vi "FTW-Endpoint-BindToListener.vi"(0 "FTW-Endpoint In":refnum<class "FTW-Endpoint.lvclass">, 5 "Address":string, 9 "Timeout":i32=1000 format="%dmsec", 11 "error in":errorcluster) -> (4 "FTW-Endpoint Out":refnum<class "FTW-Endpoint.lvclass">, 6 "Actual Address":string, 15 "error out":errorcluster)   [LabVIEW 2013, in "FTW-Endpoint.lvclass"]
uses:
  FTW-Endpoint.lvclass
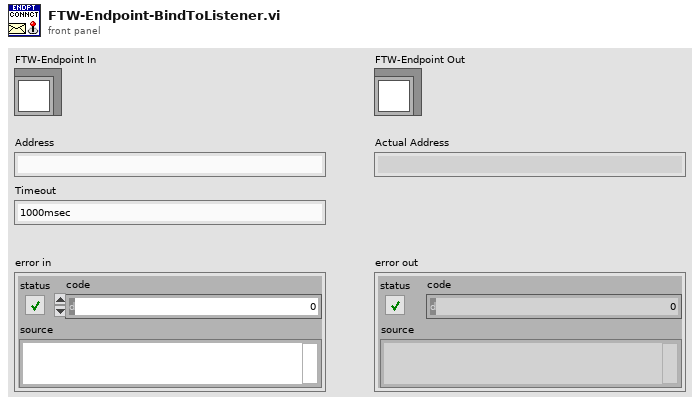
[diagram p1: front panel]
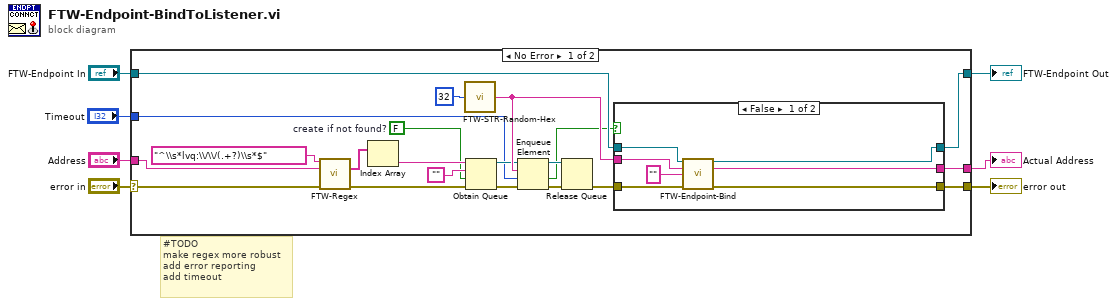
[diagram p0: block diagram]
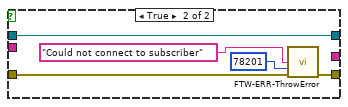
[diagram p2: hidden frame]
diagram:
  # "#TODO\nmake regex more robust\nadd error reporting\nadd timeout"
  n1 = case shown="No Error" "error in" {
    selector: "error in" -> [w26 w42]
    tunnel: [w22 w42] -> w7
    tunnel: [w21 w41] -> w6
    tunnel: "FTW-Endpoint In" -> [w27 w41]
    tunnel: "Address" -> [w18 _]
    tunnel: [w19 _] -> w2
    tunnel: "Timeout" -> [w9 _]
    frame No Error {
      w11 = FALSE  # create if not found?
      n2 = call "FTW-Regex.vi"("Regular Expression"="^\\s*lvq:\\/\\/(.+?)\\s*$" ("input string"), "Input String"=w18, "error in"=w26) -> ("Submatches"=w24:string[], "error out"=w25:errorcluster)  [unwired: 8 in, 3 out]
      n3 = Index Array(array=w24) -> (element=w23:string)  [unwired: 1 in]
      n4 = call "FTW-STR-Random-Hex.vi"("String Length"=32) -> ("Random Hex String"=w20:string)  [unwired: 3 in]
      n5 = Obtain Queue(name (unnamed)=w23, element data type="", create if not found? (T)=w11, error in (no error)=w25) -> (queue out=w14:refnum<queue>, error out=w16:errorcluster)  [unwired: 1 in, 1 out]
      n6 = Enqueue Element(queue=w14, element=w20, timeout in ms (-1)=w9, error in (no error)=w16) -> (queue out=w12:refnum<queue>, timed out?=w8:bool, error out=w15:errorcluster)
      n7 = Release Queue(queue=w12, error in (no error)=w15) -> (error out=w28:errorcluster)  [unwired: 1 in, 2 out]
      n8 = case shown="False" w8 {
        tunnel: w28 -> [w35 w39]
        tunnel: w27 -> [w34 w40]
        tunnel: [w33 w38] -> w22
        tunnel: [w32 w40] -> w21
        tunnel: w20 -> [w31 _]
        tunnel: [w30 _] -> w19
        frame False {
          n9 = call-dynamic "FTW-Endpoint-Bind.vi"("FTW Endpoint"=w34, "Endpoint Address"=w31, "Requested Identity"="", "error in"=w35) -> ("FTW Endpoint out"=w32:refnum<class "FTW-Endpoint.lvclass">, "Actual Endpoint Address"=w30:string, "error out"=w33:errorcluster)  [unwired: 8 in, 1 out]
        }
        frame True {
          n10 = call "FTW-ERR-ThrowError.vi"("Error Message"="Could not connect to subscriber", "Error Code"=78201, "error in"=w39) -> ("error out"=w38:errorcluster)  [unwired: 12 in]
        }
      }
    }
    frame Error {
    }
  }
  "FTW-Endpoint Out" <- w6
  "error out" <- w7
  "Actual Address" <- w2
